vi "stopFGV.vi"(10 "stop":bool, 11 "Enum":T1) -> (2 "stop":bool)   [LabVIEW 2017]
uses:
  typeDefs/stopfgvcontrol.ctl
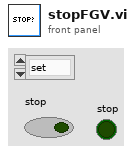
[diagram p1: front panel]
types:
  T1 = typedef "stopfgvcontrol.ctl" = enum16{"set", "get"}
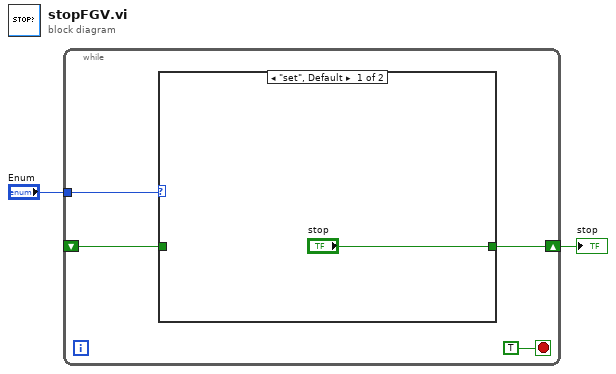
[diagram p0: block diagram]
diagram:
  n1 = while {
    tunnel: "Enum" -> [w5]
    shift-right: [w4] -> w1
    shift-left: _ -> [w3]
    stop <- TRUE stop-if-true
    n2 = case shown="\"set\", Default" w5 {
      tunnel: ["stop" w8] -> w4
      tunnel: w3 -> [_ w8]
      frame "set", Default {
      }
      frame "get" {
      }
    }
  }
  "stop" <- w1
